vi "copy.vi"(2 "Value":i32[](array[numeric]), 3 "ItemNames in":string[][](array[string])) -> (0 "val(sgnl)":i32[](array[numeric]), 1 "ItemNames out":string[][](array[string]), 4 "copyAry":string[][](array[string]))   [LabVIEW 2019]
panel:
  # "About This VI (copies highlighted portion of List and store it in \"coppery\")\n- save highlighted portion of \"ItemName in\" (2D array for LIST values) and save it as 2D array called \"copyAry\".  \n- and outputs \"ItemName out\" which is identical to \"ItemName in\""
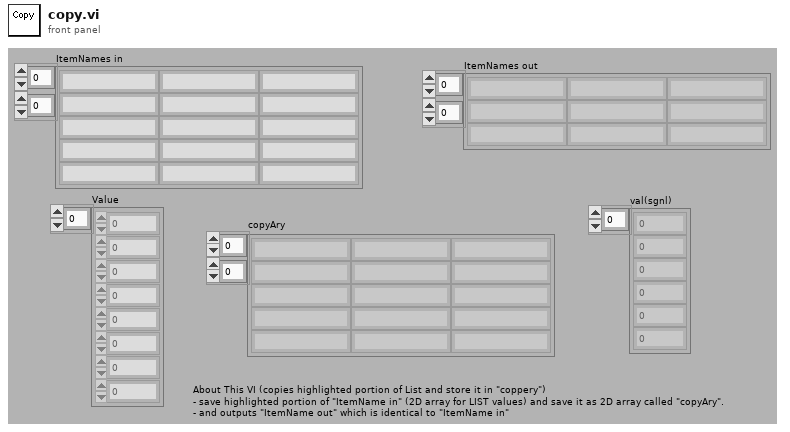
[diagram p1: front panel]
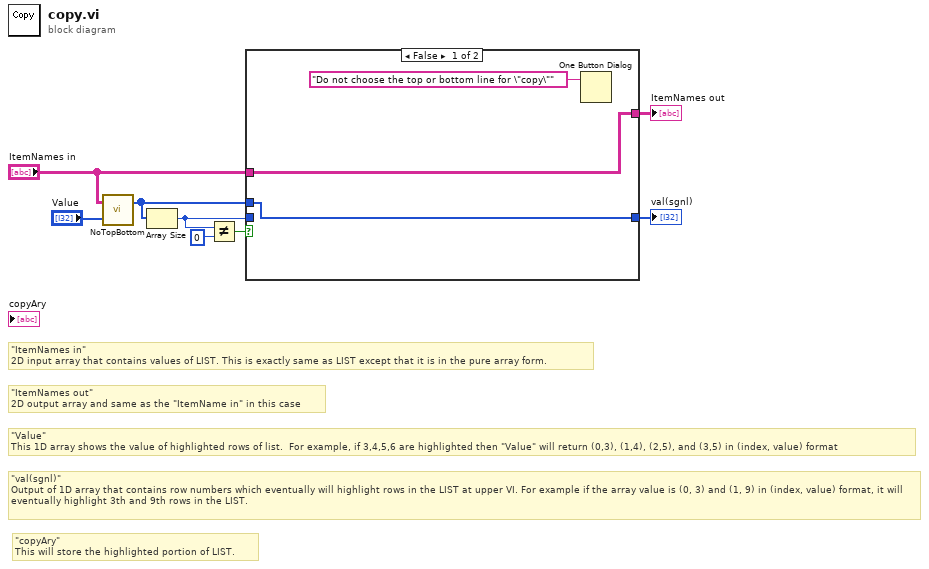
[diagram p0: block diagram]
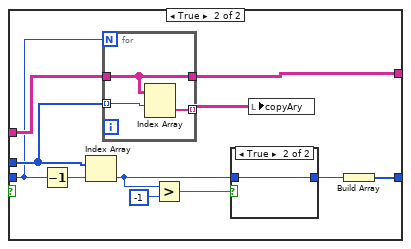
[diagram p2: hidden frame]
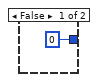
[diagram p3: hidden frame]
diagram:
  # "\"copyAry\"\nThis will store the highlighted portion of LIST."
  # "\"val(sgnl)\"\nOutput of 1D array that contains row numbers which eventually will highlight rows in the LIST at upper VI. For example if the array value is (0, 3) and (1, 9) in (index, value) format, it will eventually highlight 3th and 9th rows in the LIST."
  # "\"ItemNames out\"\n2D output array and same as the \"ItemName in\" in this case"
  # "\"ItemNames in\" \n2D input array that contains values of LIST. This is exactly same as LIST except that it is in the pure array form."
  # "\"Value\"\nThis 1D array shows the value of highlighted rows of list.  For example, if 3,4,5,6 are highlighted then \"Value\" will return (0,3), (1,4), (2,5), and (3,5) in (index, value) format"
  n1 = call "NoTopBottom.vi"("Value in"="Value", "ItemNames in"="ItemNames in") -> ("Value out"=w2:i32[])  [unwired: 1 out]
  n2 = Array Size(array=w2) -> (size(s)=w5:i32)
  n3 = Not Equal?(x=w5, y=0) -> (x != y?=w6:bool)
  n4 = case shown="False" w6 {
    tunnel: [w11 w21] -> w8
    tunnel: "ItemNames in" -> [w11 w20]
    tunnel: w2 -> [w9 w15]
    tunnel: w5 -> [_ w14]
    tunnel: [w9 w13] -> w4
    frame False {
      n5 = One Button Dialog(message="Do not choose the top or bottom line for \"copy\"") -> ()  [unwired: 1 in, 1 out]
    }
    frame True {
      n6 = Decrement(x=w14) -> (x-1=w22:i32)
      n7 = Index Array(array=w15, index=w22) -> (element=w16:i32)
      n8 = for {
        N: w14 -> [_]
        tunnel: w15 -> [w25] mode=indexing
        tunnel: [w27] -> w21
        tunnel: w20 -> [w27]
        tunnel: [w26] -> w12 mode=indexing
        n9 = Index Array(array=w27, index (row)=w25) -> (element=w26:string[])  [unwired: 1 in]
      }
      n10 = Greater?(x=w16, y=-1) -> (0:w19:bool)
      n11 = case shown="True" w19 {
        tunnel: [0 w24] -> w17
        tunnel: w16 -> [_ w24]
        frame False {
        }
        frame True {
        }
      }
      n12 = local write "copyAry"(w12) -> ()
      n13 = Build Array(w17) -> (w13:i32[])
    }
  }
  "ItemNames out" <- w8
  "val(sgnl)" <- w4
